vi "updateRowNumber.vi"(0 "Array in":refnum<vi>, 5 "Name":refnum<vi>, 7 "modeArray 2":refnum<vi>, 9 "Status 3":refnum<vi>, 11 "Description":refnum<vi>, 12 "No of channels":i32) -> ()   [LabVIEW 2013]
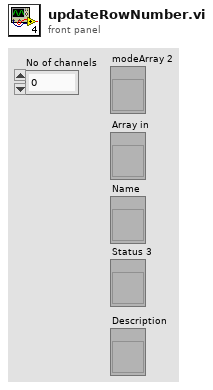
[diagram p1: front panel]
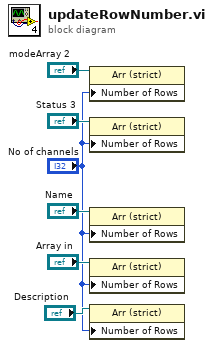
[diagram p0: block diagram]
diagram:
  n1 = property class="Arr (strict)"(reference="modeArray 2", "Number of Rows"="No of channels") -> ()  [unwired: 1 in, 2 out]
  n2 = property class="Arr (strict)"(reference="Status 3", "Number of Rows"="No of channels") -> ()  [unwired: 1 in, 2 out]
  n3 = property class="Arr (strict)"(reference="Name", "Number of Rows"="No of channels") -> ()  [unwired: 1 in, 2 out]
  n4 = property class="Arr (strict)"(reference="Array in", "Number of Rows"="No of channels") -> ()  [unwired: 1 in, 2 out]
  n5 = property class="Arr (strict)"(reference="Description", "Number of Rows"="No of channels") -> ()  [unwired: 1 in, 2 out]
